vi "Menu.Help, Add User Manual Items.vi"(5 "Ignore Errors(T)":bool=TRUE, 7 "Doc Folder":path, 8 "error in":errorcluster, 9 "Main VI":refnum<vi>, 11 "Menu Ref":refnum<k9>) -> (0 "error out":errorcluster, 1 "Tags":string[](array[string]), 2 "Paths":path[](array[path]), 3 "Menu Ref Out":refnum<k9>)   [LabVIEW 2024, in "EQMF.lvlib" / "Menu Utils.lvlib"]
uses:
  Menu Utils.lvlib
panel:
  in  "Menu Tag":string="Documentation"
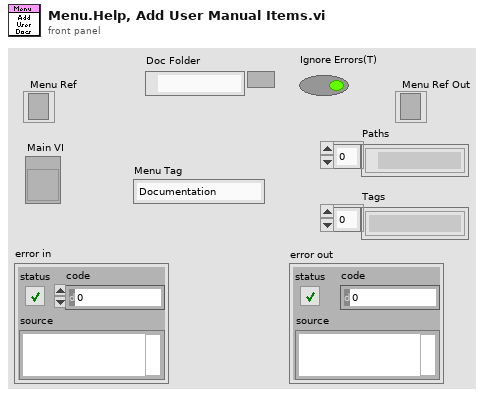
[diagram p1: front panel]
types:
  T1 = enum32{"invalid app kind", "Development System", "Run Time System", "Student Edition", "Embedded LabVIEW", "Evaluation", "Custom"}
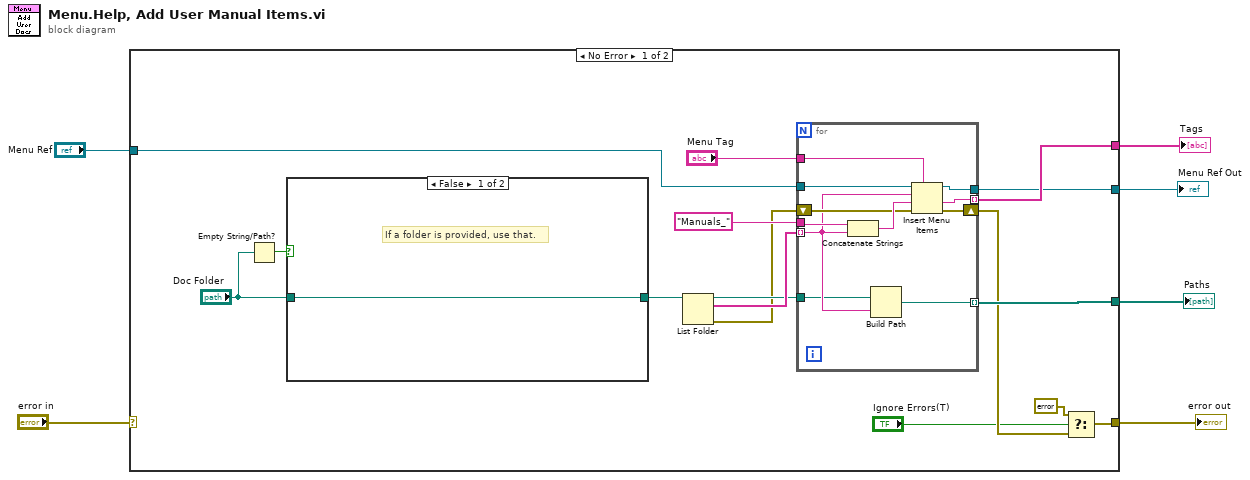
[diagram p0: block diagram]
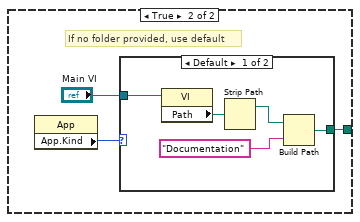
[diagram p2: hidden frame]
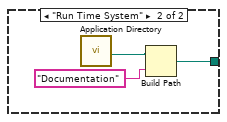
[diagram p3: hidden frame]
diagram:
  n1 = case shown="No Error" "error in" {
    selector: "error in" -> [_ w47]
    tunnel: [w21 _] -> w6
    tunnel: [w20 w46] -> w5
    tunnel: [w10 w47] -> w4
    tunnel: [w17 _] -> w3
    tunnel: "Menu Ref" -> [w11 w46]
    frame No Error {
      n2 = Empty String/Path?(string/path="Doc Folder") -> (empty?=w13:bool)
      n3 = case shown="False" w13 {
        tunnel: [w23 w24] -> w14
        tunnel: "Doc Folder" -> [w23 _]
        frame False {
          # "If a folder is provided, use that."
        }
        frame True {
          # "If no folder provided, use default"
          n4 = property class="App"() -> ("App.Kind"=w26:T1)  [unwired: 2 in, 2 out]
          n5 = case shown="Default" w26 {
            tunnel: [w28 w33] -> w24
            tunnel: "Main VI" -> [w30 _]
            frame Default {
              n6 = property class="VI"(reference=w30) -> ("Path"=w31:path)  [unwired: 1 in, 2 out]
              n7 = Strip Path(path=w31) -> (stripped path=w29:path)  [unwired: 1 out]
              n8 = Build Path(base path=w29, name or relative path="Documentation") -> (appended path=w28:path)
            }
            frame "Run Time System" {
              n9 = call <vilib>:"Application Directory.vi"() -> ("Application Directory"=w34:path)
              n10 = Build Path(base path=w34, name or relative path="Documentation") -> (appended path=w33:path)
            }
          }
        }
      }
      n11 = List Folder(path=w14) -> (path out=w18:path, filenames=w19:string[], error out=w15:errorcluster)  [unwired: 3 in, 1 out]
      n12 = for {
        tunnel: w11 -> [w45]
        tunnel: "Menu Tag" -> [w44]
        tunnel: "Manuals_" -> [w43]
        tunnel: w19 -> [w37] mode=indexing
        tunnel: [w41] -> w21 mode=indexing
        tunnel: [w40] -> w20
        shift-right: [w38] -> w9
        shift-left: w15 -> [w39]
        tunnel: w18 -> [w36]
        tunnel: [w35] -> w17 mode=indexing
        n13 = Concatenate Strings(w43, w37) -> (w42:string)
        n14 = Build Path(base path=w36, name or relative path=w37) -> (appended path=w35:path)
        n15 = Insert Menu Items(5:w44, 6:w39, 7:w42, 8:w37, 9:w45) -> (0:w38:errorcluster, 1:w41:string, 3:w40:refnum<k9>)  [unwired: 1 in]
      }
      n16 = Select(t=errorcluster {"status"=FALSE, "code"=0, "source"=""} ("error constant"), s="Ignore Errors(T)", f=w9) -> (s? t:f=w10:errorcluster)
    }
    frame Error {
    }
  }
  "error out" <- w4
  "Menu Ref Out" <- w5
  "Paths" <- w3
  "Tags" <- w6
